vi "myRIO_BRig_RT_dataBlock_T2R__L.vi"() -> (2 "output_T2R__L":i32)   [LabVIEW 2014]
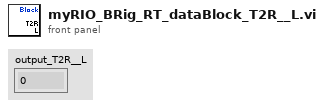
[diagram p1: front panel]
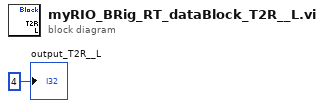
[diagram p0: block diagram]
diagram:
  "output_T2R__L" <- 4 ("output_iBlock")
